vi "DisconnectAndReleaseAllStages.vi"(8 "error in (no error)":errorcluster, 11 "Config In":T1 {"Hardware Configuration"."Lasers Configuration"."SettingValues"."785 Power" format="%.1f"; "Hardware Configuration"."Lasers Configuration"."SettingValues"."647 Power" format="%.1f"; "Hardware Configuration"."Lasers Configuration"."SettingValues"."561 Power" format="%.1f"; "Hardware Configuration"."Lasers Configuration"."SettingValues"."532 Power" format="%.1f"; "Hardware Configuration"."Lasers Configuration"."SettingValues"."488 Power" format="%.1f"; "Hardware Configuration"."Lasers Configuration"."SettingValues"."405 Power" format="%.1f"}) -> (0 "error out":errorcluster, 3 "Config Out":T1 {"Hardware Configuration"."Lasers Configuration"."SettingValues"."785 Power" format="%.1f"; "Hardware Configuration"."Lasers Configuration"."SettingValues"."647 Power" format="%.1f"; "Hardware Configuration"."Lasers Configuration"."SettingValues"."561 Power" format="%.1f"; "Hardware Configuration"."Lasers Configuration"."SettingValues"."532 Power" format="%.1f"; "Hardware Configuration"."Lasers Configuration"."SettingValues"."488 Power" format="%.1f"; "Hardware Configuration"."Lasers Configuration"."SettingValues"."405 Power" format="%.1f"})   [LabVIEW 2019]
uses:
  Settings/Settings.ctl
  Support/Hardware Configuration.ctl
  Support/Camera Configuration.ctl
  D:/SDK/PMQI-LabViewSamples/Examples/Dependencies/PVCamNET.dll
  <vilib>/vision/Image Controls.llb/IMAQ Image.ctl
  <vilib>/userdefined/High Color/IMAQdx.ctl
  E:/DevHardSoftware/MMicroscopy/HardwareAdapter/Lasers/Dependencies/Oxxius_Boxx.dll
  Lasers/Dependencies/Oxxius_Boxx.dll
  Logging/Logging Configuration.ctl
  controls/UI Configuration.ctl
  controls/CallBack Refs.ctl
  Dependencies/Madlib.dll
  Dependencies/MicroDrive.dll
  Dependencies/TIRF-Lock.dll
  Logging/Logging.lvlib
  Settings/Settings.lvlib
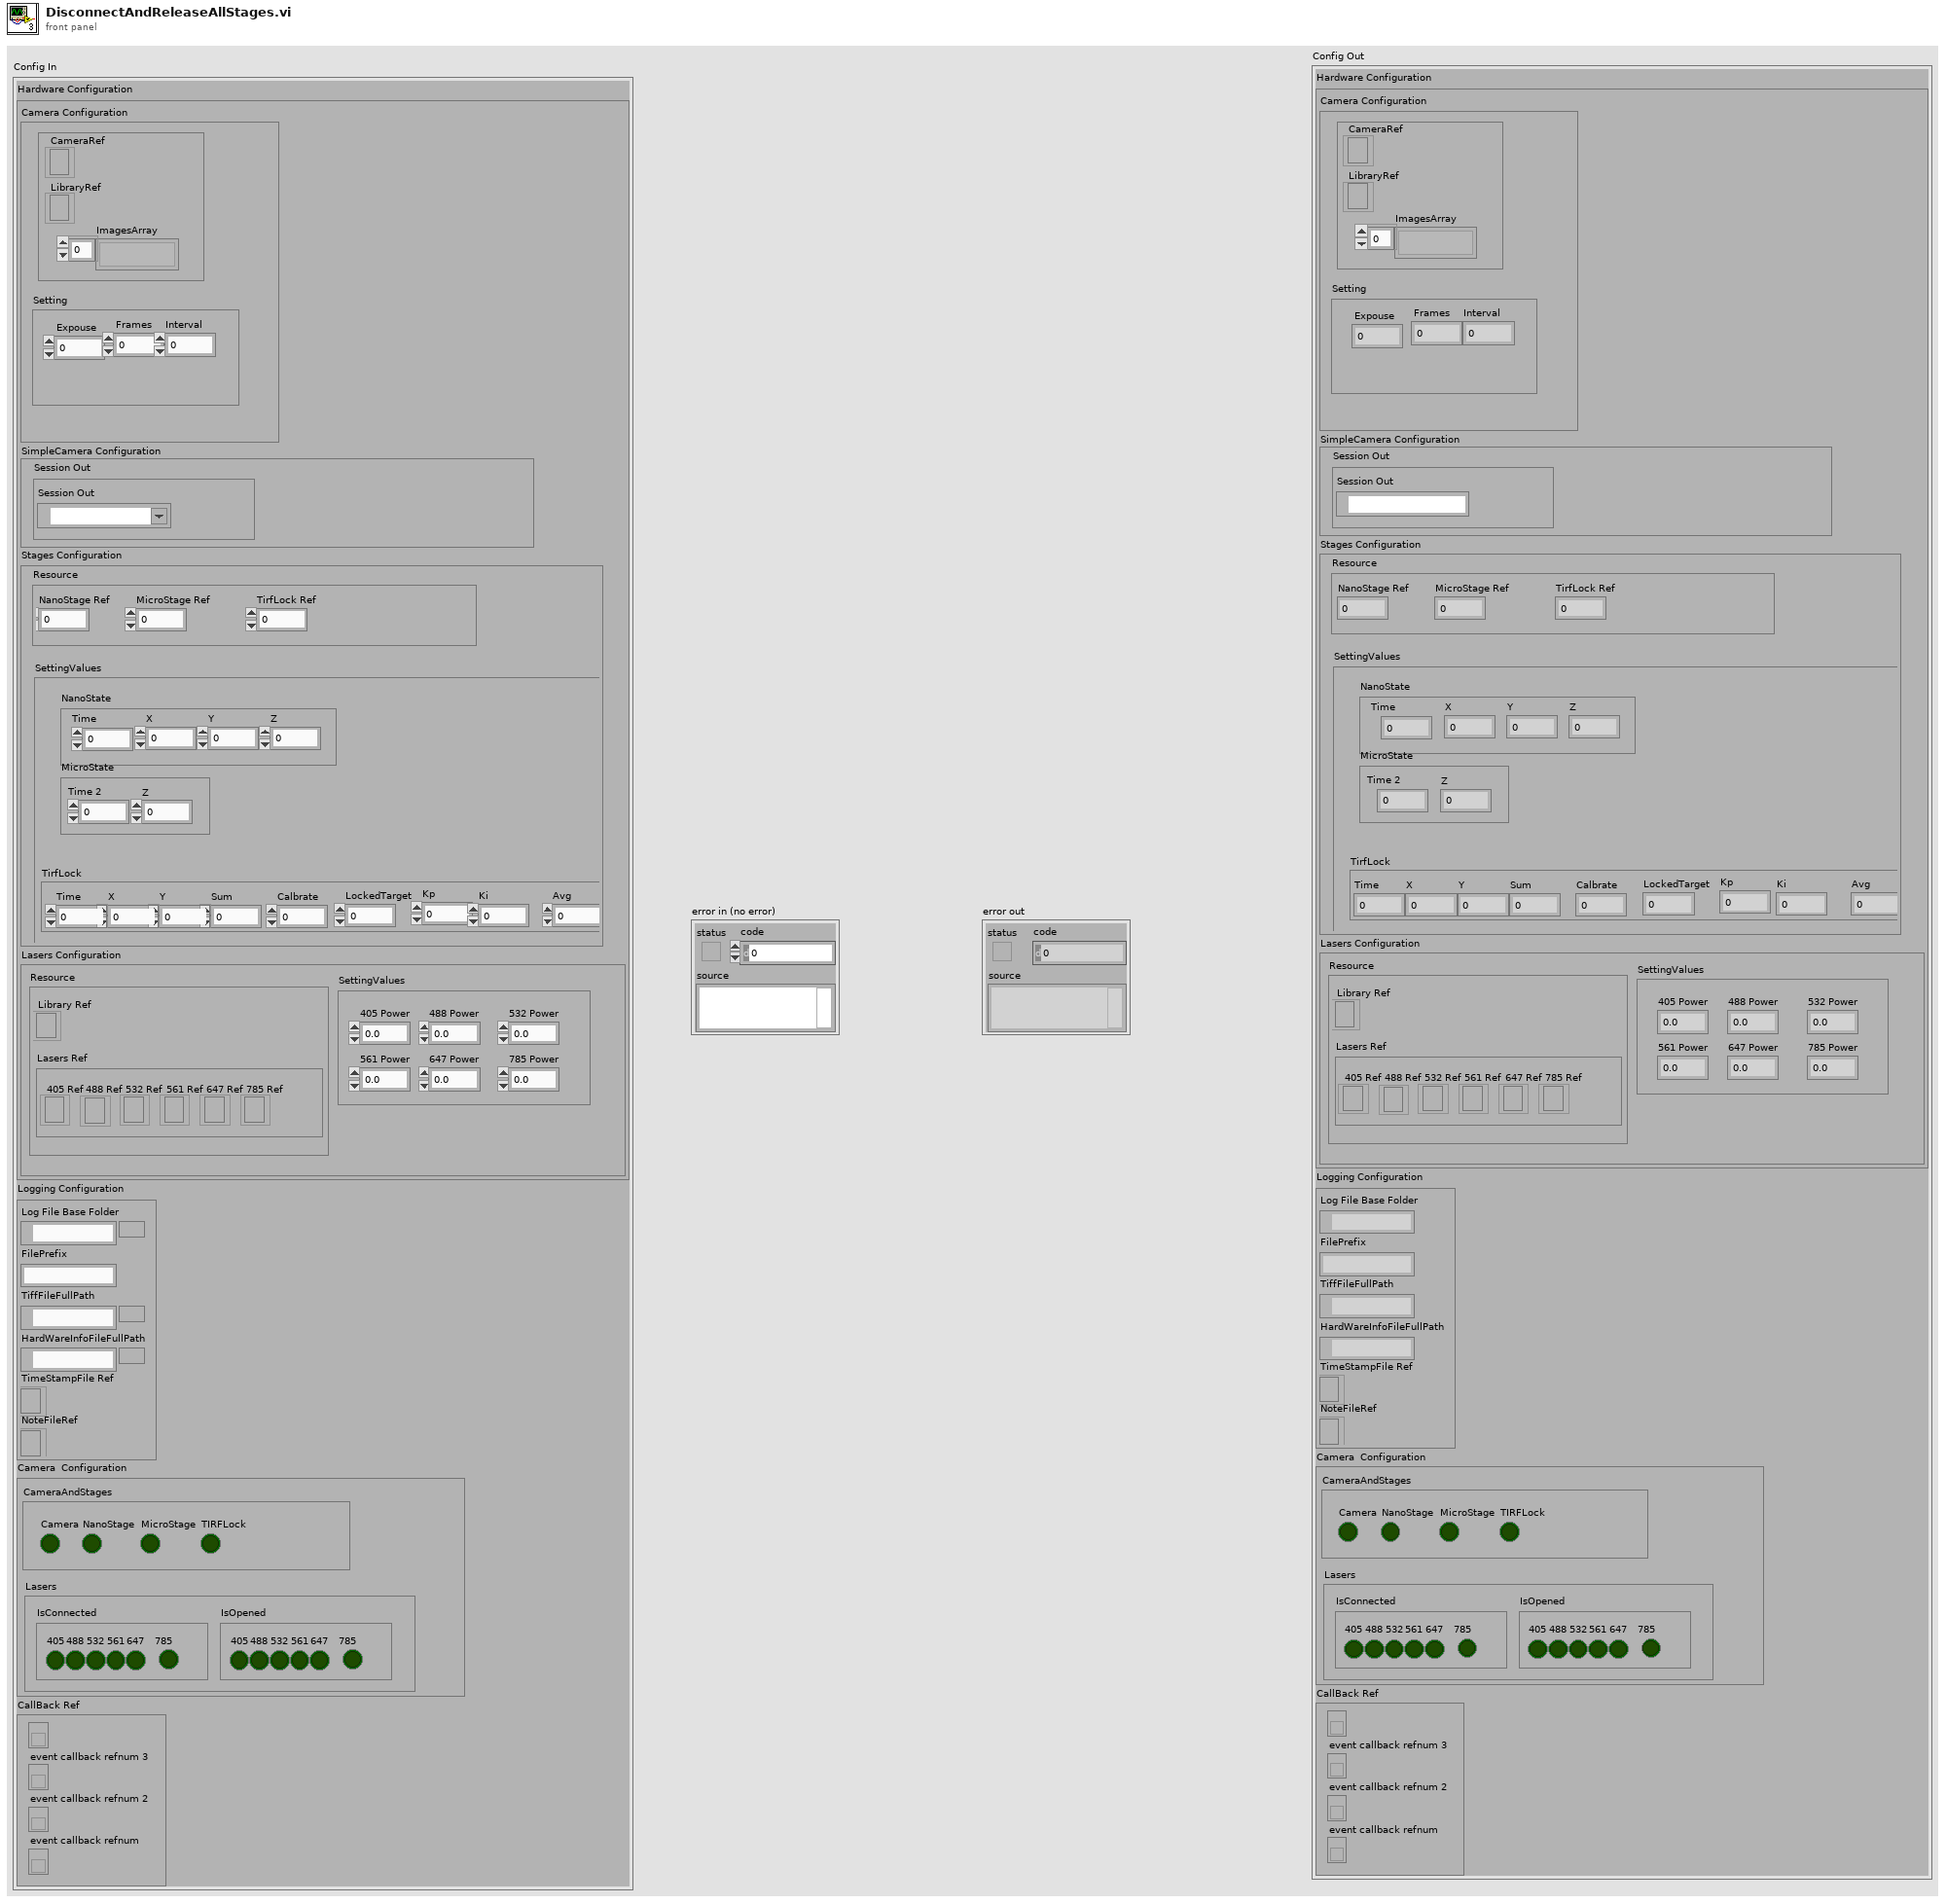
[diagram p1: front panel]
types:
  T1 = typedef "Settings.lvlib/Settings.ctl" = cluster{"Hardware Configuration":T2, "Logging Configuration":T6, "HardWare Status":cluster{"CameraAndStages":T7, "Lasers":cluster{"IsConnected":cluster{"405":bool, "488":bool, "532":bool, "561":bool, "647":bool, "785":bool}, "IsOpened":cluster{"405":bool, "488":bool, "532":bool, "561":bool, "647":bool, "785":bool}}}, "CallBack Ref":T8}
  T2 = typedef "Hardware Configuration.ctl" = cluster{"Camera Configuration":T3, "SimpleCamera Configuration":cluster{"Resource":cluster{"Session Out":T5}}, "Stages Configuration":cluster{"Resource":cluster{"NanoStage Ref":i32, "MicroStage Ref":i32, "TirfLock Ref":i32}, "SettingValues":cluster{"NanoState":cluster{"Time":dbl, "X":dbl, "Y":dbl, "Z":dbl}, "MicroState":cluster{"Time 2":dbl, "Z":dbl}, "TirfLock":cluster{"Time":dbl, "X":dbl, "Y":dbl, "Sum":dbl, "Calbrate":dbl, "LockedTarget":dbl, "Kp":dbl, "Ki":dbl, "Avg":dbl}}}, "Lasers Configuration":cluster{"SettingValues":cluster{"405 Power":sgl, "488 Power":sgl, "532 Power":sgl, "561 Power":sgl, "647 Power":sgl, "785 Power":sgl}, "Resource":cluster{"Library Ref":refnum<k24>, "Lasers Ref":cluster{"405 Ref":refnum<k24>, "488 Ref":refnum<k24>, "532 Ref":refnum<k24>, "561 Ref":refnum<k24>, "647 Ref":refnum<k24>, "785 Ref":refnum<k24>}}}}
  T3 = typedef "Camera Configuration.ctl" = cluster{"Setting":cluster{"Expouse":dbl, "Frames":dbl, "Interval":dbl}, "Resource":cluster{"CameraRef":refnum<k24>, "LibraryRef":refnum<k24>, "ImagesArray":T4[]}}
  T4 = typedef "IMAQ Image.ctl" = refnum<image>
  T5 = typedef "IMAQdx.ctl" = refnum<k21>
  T6 = typedef "Logging.lvlib/Logging Configuration.ctl" = cluster{"Log File Base Folder":path, "FilePrefix":string, "TiffFileFullPath":path, "HardWareInfoFileFullPath":path, "TimeStampFile Ref":refnum<file>, "NoteFileRef":refnum<file>}
  T7 = typedef "UI Configuration.ctl" = cluster{"Camera":bool, "NanoStage":bool, "MicroStage":bool, "TIRFLock":bool}
  T8 = typedef "CallBack Refs.ctl" = cluster{"event callback refnum":refnum<k27>, "event callback refnum 2":refnum<k27>, "event callback refnum 3":refnum<k27>, "event callback refnum 4":refnum<k27>}
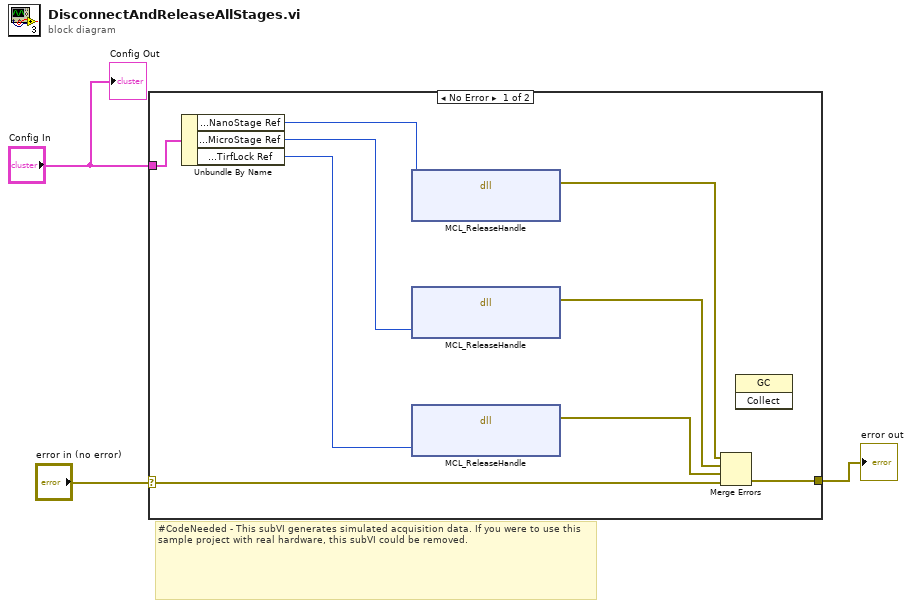
[diagram p0: block diagram]
diagram:
  # "#CodeNeeded - This subVI generates simulated acquisition data. If you were to use this sample project with real hardware, this subVI could be removed."
  n1 = case shown="No Error" "error in (no error)" {
    selector: "error in (no error)" -> [w7 w13]
    tunnel: [w8 w13] -> w2
    tunnel: "Config In" -> [w12 _]
    frame No Error {
      n2 = Unbundle By Name(w12) -> ("Hardware Configuration.Stages Configuration.Resource.NanoStage Ref"=w11:i32, "Hardware Configuration.Stages Configuration.Resource.MicroStage Ref"=w10:i32, "Hardware Configuration.Stages Configuration.Resource.TirfLock Ref"=w9:i32)
      n3 = dll-call lib="E:/DevHardSoftware/MMicroscopy/HardwareAdapter/Stages/Dependencies/Madlib.dll" fn="MCL_ReleaseHandle"("handle"=w11) -> (error out=w4:errorcluster)  [unwired: 4 in, 2 out]
      n4 = dll-call lib="E:/DevHardSoftware/MMicroscopy/HardwareAdapter/Stages/Dependencies/MicroDrive.dll" fn="MCL_ReleaseHandle"("handle"=w10) -> (error out=w5:errorcluster)  [unwired: 4 in, 2 out]
      n5 = dll-call lib="E:/DevHardSoftware/MMicroscopy/HardwareAdapter/Stages/Dependencies/TIRF-Lock.dll" fn="MCL_ReleaseHandle"("handle"=w9) -> (error out=w6:errorcluster)  [unwired: 4 in, 2 out]
      n6 = Merge Errors(w4, w5, w6, w7) -> (w8:errorcluster)
      n7 = invoke class="GC" method="Collect"() -> ()  [unwired: 3 in, 3 out]
    }
    frame Error {
    }
  }
  "error out" <- w2
  "Config Out" <- "Config In"
